vi "hasField.vi"(8 "error in (no error)":errorcluster, 10 "Name in":string, 11 "IStruct in":refnum<class "IStruct.lvclass">) -> (0 "error out":errorcluster, 3 "IStruct out":refnum<class "IStruct.lvclass">)   [LabVIEW 2022 SP3, in "openDAQ.lvlib" / "daqCoreTypes.lvlib" / "IStruct.lvclass"]
uses:
  <instrlib>/openDAQ/Public/Classes/daqCoreTypes/IStruct/IStruct.lvclass
  <instrlib>/openDAQ/Public/Classes/daqCoreTypes/IStruct/IStruct.lvclass/IStruct.ctl
  <instrlib>/openDAQ/Public/Classes/daqCoreTypes/IString/IString.lvclass
  <instrlib>/openDAQ/Binaries/Windows/x86/copendaq32.dll
panel:
  out "Contains?":bool
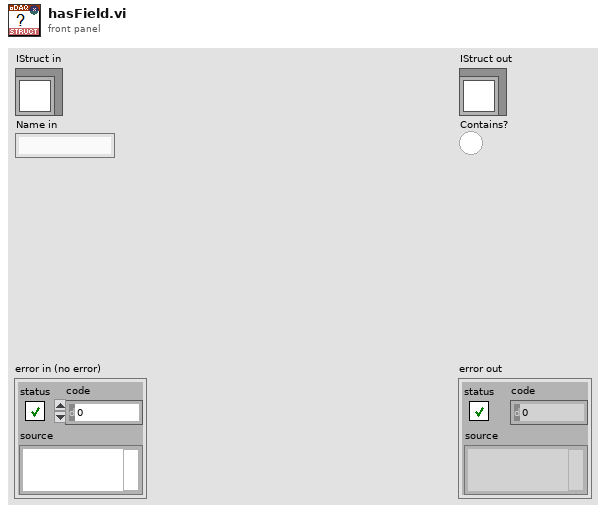
[diagram p1: front panel]
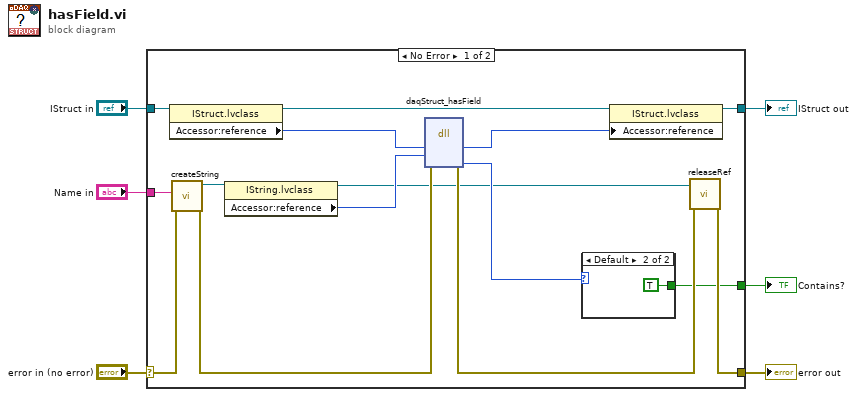
[diagram p0: block diagram]
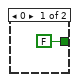
[diagram p2: hidden frame]
diagram:
  n1 = case shown="No Error" "error in (no error)" {
    selector: "error in (no error)" -> [w14 w25]
    tunnel: [w9 w25] -> w5
    tunnel: [w17 w24] -> w3
    tunnel: "IStruct in" -> [w20 w24]
    tunnel: "Name in" -> [w15 _]
    tunnel: [w7 _] -> w1
    frame No Error {
      n2 = property class="IStruct.lvclass"(reference=w20) -> (reference out=w18:refnum<class "IStruct.lvclass">, "Accessor:reference"=w19:i64)  [unwired: 1 in, 1 out]
      n3 = call <instrlib>:"createString.vi"("error in (no error)"=w14, "String"=w15) -> ("error out"=w13:errorcluster, "IString out"=w12:refnum<class "IString.lvclass">)  [unwired: 8 in]
      n4 = property class="IString.lvclass"(reference=w12) -> (reference out=w8:refnum<class "IString.lvclass">, "Accessor:reference"=w11:i64)  [unwired: 1 in, 1 out]
      n5 = dll-call lib="C:/Program Files (x86)/National Instruments/LabVIEW 2022/instr.lib/openDAQ/Binaries/Windows/x86/copendaq*.*" fn="daqStruct_hasField"(error in=w13, "struct"=w19, "name"=w11) -> (error out=w10:errorcluster, "struct"=w16:i64, "contains"=w21:i64)  [unwired: 5 in, 1 out]
      n6 = case shown="Default" w21 {
        tunnel: [FALSE TRUE] -> w7
        frame 0 {
        }
        frame Default {
        }
      }
      n7 = property class="IStruct.lvclass"(reference=w18, "Accessor:reference"=w16) -> (reference out=w17:refnum<class "IStruct.lvclass">)  [unwired: 1 in, 1 out]
      n8 = call-dynamic "releaseRef.vi"("error in (no error)"=w10, "IBaseObject in"=w8) -> ("error out"=w9:errorcluster)  [unwired: 9 in]
    }
    frame Error {
    }
  }
  "error out" <- w5
  "IStruct out" <- w3
  "Contains?" <- w1
